vi "Write to txt.vi"(8 "error in":errorcluster, 11 "Input string":string) -> (0 "error out":errorcluster)   [LabVIEW 2017, in "Akwizycja.lvlib"]
uses:
  Akwizycja.lvlib
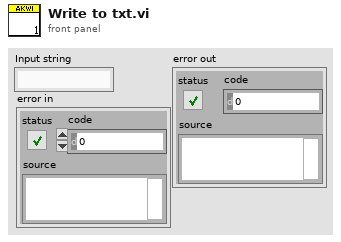
[diagram p1: front panel]
types:
  T1 = enum16{"open", "replace", "create", "open or create", "replace or create", "replace or create with confirmation"}
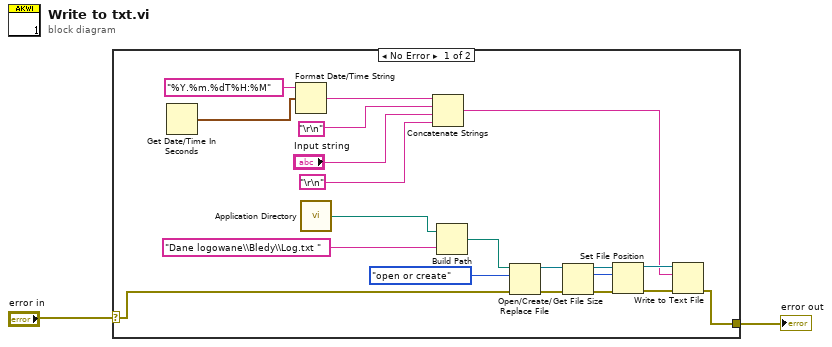
[diagram p0: block diagram]
diagram:
  n1 = case shown="No Error" "error in" {
    selector: "error in" -> [w4 w23]
    tunnel: [w3 w23] -> w1
    frame No Error {
      n2 = Get Date/Time In Seconds() -> (seconds since 1Jan1904=w12:timestamp)
      n3 = Format Date/Time String(time format string (%c)="%Y.%m.%dT%H:%M", seconds (now)=w12) -> (date/time string=w7:string)  [unwired: 1 in]
      n4 = call <vilib>:"Application Directory.vi"() -> ("Application Directory"=w20:path)
      n5 = Concatenate Strings(w7, "\r\n", "Input string", "\r\n") -> (w9:string)
      n6 = Build Path(base path=w20, name or relative path="Dane logowane\\Bledy\\Log.txt ") -> (appended path=w22:path)
      n7 = Open/Create/Replace File(file path (use dialog)=w22, error in=w4, operation (0:open)=T1."open or create") -> (refnum out=w18:refnum<file>, error out=w17:errorcluster)  [unwired: 3 in, 1 out]
      n8 = Get File Size(file=w18, error in=w17) -> (refnum out=w14:refnum<file>, size (in bytes)=w11:i64, 0:w16:errorcluster)
      n9 = Set File Position(offset (in bytes) (0)=w11, refnum=w14, error in=w16) -> (refnum out=w13:refnum<file>, error out=w15:errorcluster)  [unwired: 1 in]
      n10 = Write to Text File(file (use dialog)=w13, text=w9, error in=w15) -> (error out=w3:errorcluster)  [unwired: 1 in, 2 out]
    }
    frame Error {
    }
  }
  "error out" <- w1
